vi "Ouptut_Sound_trace_ph.vi"() -> (5 "Plug in titles":string[](array[string]), 7 "Plug in values":string[](array[string]))   [LabVIEW 2011]
doc: "This VI demonstrates how to output continuous sound using SO Set Num Buffers. This example is available only on Windows."
uses:
  <vilib>/sound2/lvsound2.llb/Sound Data Format.ctl
  <vilib>/sound2/lvsound2.llb/Sampling Mode.ctl
  Globals/Meas_global.vi
  <vilib>/Utility/file.llb/Read From Spreadsheet File (DBL).vi
  <vilib>/sound2/lvsound2.llb/Sound Output Write (DBL Single).vi
  <vilib>/measure/NI_MABase.lvlib
panel:
  out "Trace Length (s)":dbl
  in  "Dwell Time (s)":dbl=0.1
  in  "Desired Amplitudes":dbl[](array[numeric])=[0.1, 0.15, 0.25]
  in  "Desired Frequencies":dbl[](array[numeric])=[1000.0, 2000.0, 2500.0, 3500.0]
  in  "Number of Cycles":i32=100
  out "Numeric":i32=4
  in  "Device ID":u32
  in  "Sound Format":T1={"sample rate (S/s)"=44100.0, "number of channels"=1, "bits per sample"=16}
  in  "Generate Sine output":bool=TRUE
  in  "Path":path
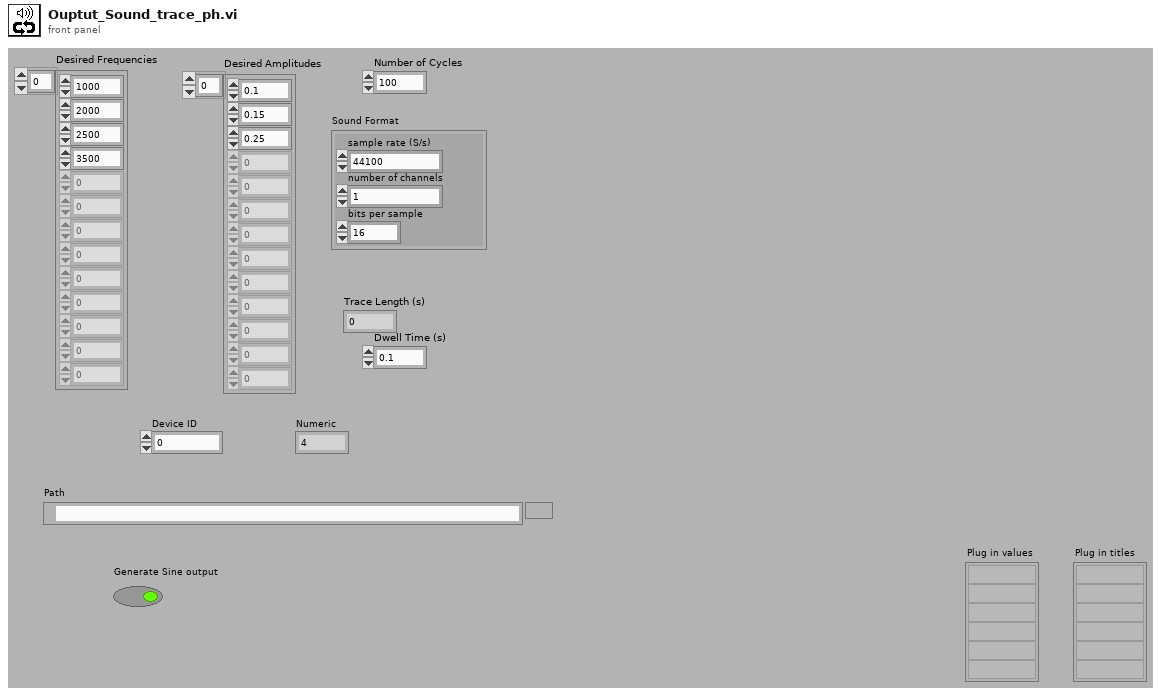
[diagram p1: front panel]
types:
  T1 = typedef "Sound Data Format.ctl" = cluster{"sample rate (S/s)":dbl, "number of channels":i32, "bits per sample":i32}
  T2 = typedef "Post_Process.ctl" = enum16{"Take New Data", "Post Process Raw Data File"}
  T3 = typedef "Sampling Mode.ctl" = i32
  T4 = typedef "Sound Output Task ID.ctl" = u32
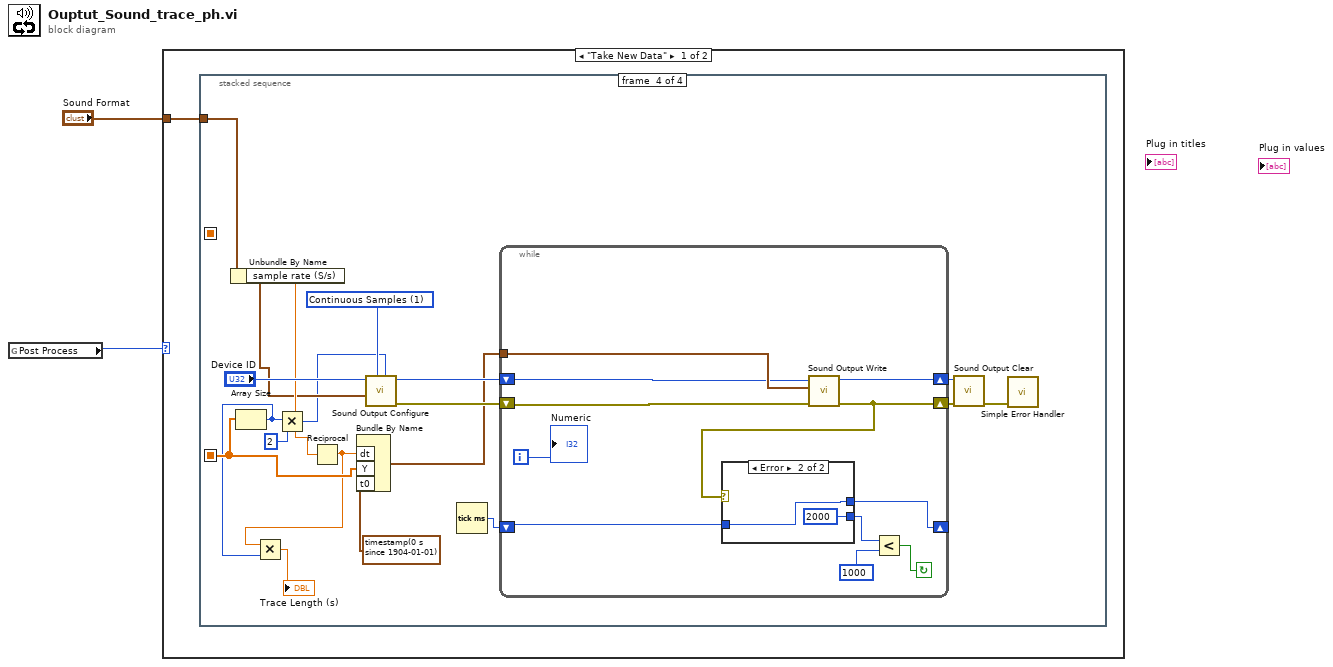
[diagram p0: block diagram]
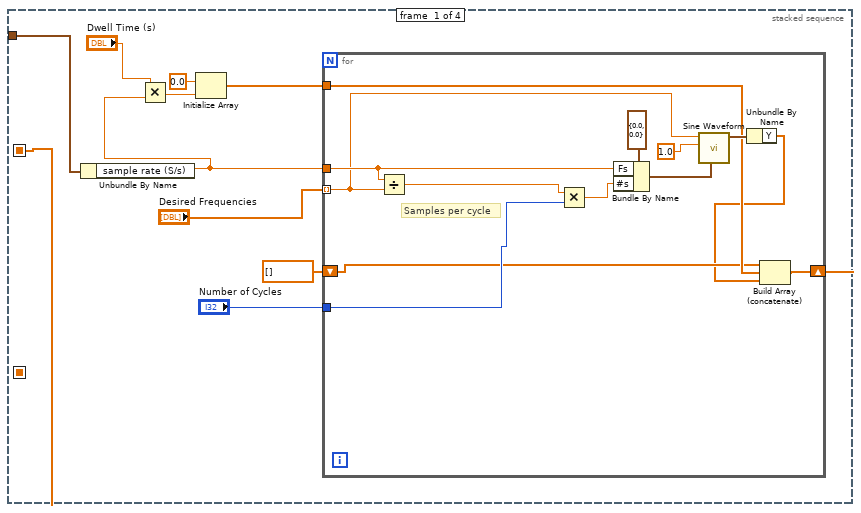
[diagram p2: hidden frame]
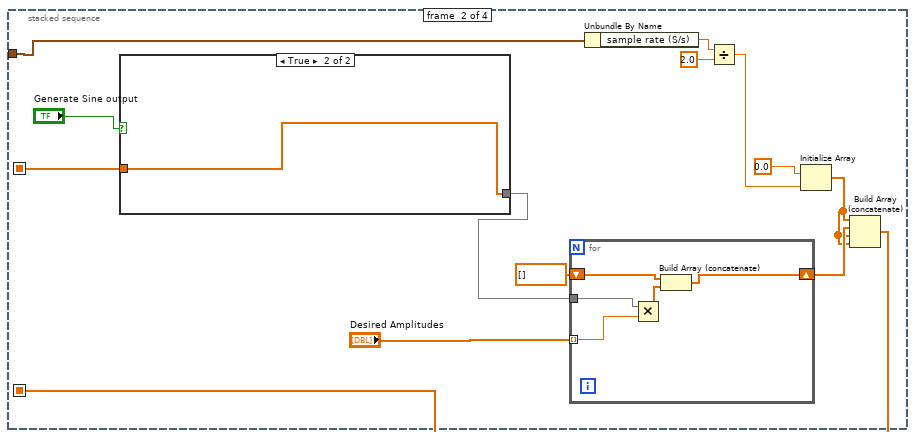
[diagram p3: hidden frame]
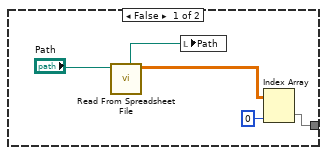
[diagram p4: hidden frame]
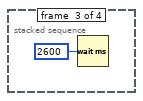
[diagram p5: hidden frame]
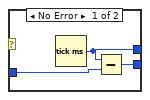
[diagram p6: hidden frame]
diagram:
  n1 = global read "Meas_global.vi" "Post Process"() -> (w2:T2)
  n2 = case shown="\"Take New Data\"" w2 {
    tunnel: "Sound Format" -> [w3 _]
    frame "Take New Data" {
      n3 = stacked-sequence {
        seq-local: [_ w32 _ _] -> [_ _ _ w57]
        seq-local: [w4 _ _ _] -> [_ w34 _ _]
        tunnel: w3 -> [w13 w31 _ w59]
        frame #0 {
          n4 = Unbundle By Name(w13) -> ("sample rate (S/s)"=w10:dbl)
          n5 = Multiply(x="Dwell Time (s)", y=w10) -> (x*y=w8:dbl)
          n6 = Initialize Array(0.0 ("element"), w8) -> (w6:dbl[])
          n7 = for {
            tunnel: w10 -> [w25]
            tunnel: "Desired Frequencies" -> [w15] mode=indexing
            tunnel: "Number of Cycles" -> [w24]
            shift-right: [w16] -> w4
            shift-left: dbl[] [] -> [w17]
            tunnel: w6 -> [w18]
            # "Samples per cycle"
            n8 = Divide(x=w25, y=w15) -> (x/y=w21:dbl)
            n9 = Multiply(x=w21, y=w24) -> (x*y=w23:dbl)
            n10 = Bundle By Name(cluster=cluster{"Fs":dbl, "#s":dbl} {"Fs"=0.0, "#s"=0.0} ("sampling info"), "Fs"=w25, "#s"=w23) -> (w20:cluster{"Fs":dbl, "#s":dbl})
            n11 = call <vilib>:"Sine Waveform.vi"("sampling info"=w20, "amplitude"=1.0, "frequency"=w15) -> ("signal out"=w19:waveform(dbl))  [unwired: 7 in, 1 out]
            n12 = Unbundle By Name(w19) -> ("Y"=w14:dbl[])
            n13 = Build Array (concatenate)(w17, w18, w14) -> (w16:dbl[])
          }
        }
        frame #1 {
          n14 = case shown="True" "Generate Sine output" {
            tunnel: [w40 w45] -> w35
            tunnel: w34 -> [_ w45]
            frame False {
              n15 = call-poly <vilib>:"Read From Spreadsheet File.vi"("file path (dialog if empty)"="Path") -> ("all rows"=w44:dbl[][], "new file path (Not A Path if cancelled)"=w41:path)  [unwired: 3 in, 6 out]
              n16 = local write "Path"(w41) -> ()
              n17 = Index Array(array=w44, index (col)=0 ("disabled index (col)")) -> (element=w40:dbl[])  [unwired: 1 in]
            }
            frame True {
            }
          }
          n18 = for {
            shift-right: [w49] -> w36
            shift-left: dbl[] [] -> [w50]
            tunnel: w35 -> [w48]
            tunnel: "Desired Amplitudes" -> [w46] mode=indexing
            n19 = Multiply(x=w48, y=w46) -> (x*y=w47:dbl[])
            n20 = Build Array (concatenate)(w50, w47) -> (w49:dbl[])
          }
          n21 = Unbundle By Name(w31) -> ("sample rate (S/s)"=w30:dbl)
          n22 = Divide(x=w30, y=2.0) -> (x/y=w28:dbl)
          n23 = Initialize Array(0.0 ("x"), w28) -> (w27:dbl[])
          n24 = Build Array (concatenate)(w27, w36, w27, w27) -> (w32:dbl[])
        }
        frame #2 {
          n25 = Wait (ms)(milliseconds to wait=u32 2600) -> ()  [unwired: 1 out]
        }
        frame #3 {
          w64 = T3 1 items=["Finite Samples", "Continuous Samples"] ("sample mode")
          n26 = Unbundle By Name(w59) -> ("sample rate (S/s)"=w61:dbl)
          n27 = Array Size(array=w57) -> (size(s)=w53:i32)
          n28 = Multiply(x=w53, y=2) -> (x*y=w56:i32)
          n29 = Reciprocal(x=w61) -> (1/x=w54:dbl)
          n30 = Multiply(x=w54, y=w53) -> (x*y=→"Trace Length (s)":dbl)
          n31 = Bundle By Name("dt"=w54, "Y"=w57, "t0"=timestamp(0 s since 1904-01-01)) -> (w60:waveform(dbl))  [unwired: 1 out]
          n32 = call <vilib>:"Sound Output Configure.vi"("number of samples/ch"=w56, "sample mode"=w64, "sound format"=w59, "device ID"="Device ID") -> ("error out"=w69:errorcluster, "task ID"=w68:T4)  [unwired: 6 in]
          n33 = Tick Count (ms)() -> (millisecond timer value=w58:u32)
          n34 = while {
            shift-right: [w70] -> w67
            shift-left: w69 -> [w77]
            shift-right: [w80] -> w66
            shift-left: w68 -> [w76]
            tunnel: w60 -> [w78]
            shift-right: [w74] -> _
            shift-left: w58 -> [w75]
            i -> [w79]
            stop <- w71 continue-if-true
            n35 = call-poly <vilib>:"Sound Output Write.vi"("error in (no error)"=w77, "data"=w78, "task ID"=w76) -> ("error out"=w70:errorcluster, "task ID out"=w80:T4)  [unwired: 7 in]
            n36 = case shown="Error" w70 {
              tunnel: w75 -> [w83 w85]
              tunnel: [w82 w85] -> w74
              tunnel: [w81 u32 2000] -> w72
              frame No Error {
                n37 = Tick Count (ms)() -> (millisecond timer value=w82:u32)
                n38 = Subtract(x=w82, y=w83) -> (x-y=w81:u32)
              }
              frame Error {
              }
            }
            n39 = Less?(x=w72, y=u32 1000) -> (x < y?=w71:bool)
            "Numeric" <- w79
          }
          n40 = call <vilib>:"Sound Output Clear.vi"("error in (no error)"=w67, "task ID"=w66) -> ("error out"=w63:errorcluster)  [unwired: 9 in]
          n41 = call <vilib>:"Simple Error Handler.vi"("error in (no error)"=w63) -> ()  [unwired: 4 in, 5 out]
        }
      }
    }
    frame "Post Process Raw Data File" {
    }
  }
